vi "Flatten I2C Linux Header.vi"(8 "error in (no error)":errorcluster, 9 "Flattened Data in":u8[](array[numeric])=[0, 0, 0, 0, 0, 0, 0, 0] format="%.0x", 10 "I2C Linux Header in":T1, 11 "pcap Parse and Build in":refnum<class "pcap Parse and Build.lvclass">) -> (0 "error out":errorcluster, 1 "Flattened Data out":u8[](array[numeric])=[0, 0, 0, 0, 0, 0, 0, 0, 1, 2, 3, 4, 5], 2 "I2C Linux Header out":T1, 3 "pcap Parse and Build out":refnum<class "pcap Parse and Build.lvclass">)   [LabVIEW 2021, in "pcap Parse and Build.lvclass"]
uses:
  pcap Parse and Build.lvclass
  pcap Parse and Build.lvclass/pcap Parse and Build.ctl
  e4177ba7-55c0-4140-bea2-15e5e44a53d0.vi
  Typedef/I2C Linux Header.ctl
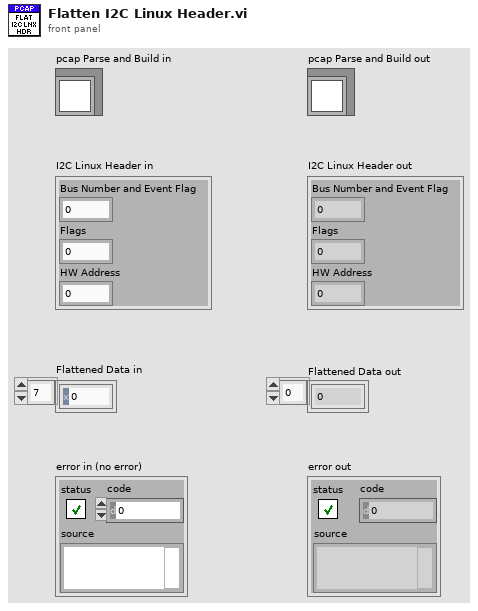
[diagram p1: front panel]
types:
  T1 = typedef "pcap Parse and Build.lvclass/I2C Linux Header.ctl" = cluster{"Bus Number and Event Flag":u8, "Flags":u32, "HW Address":u8}
  T2 = typedef "DataTypes_CIF_U.lvlib/Endian.ctl" = enum16{"Little Endian", "Big Endian"}
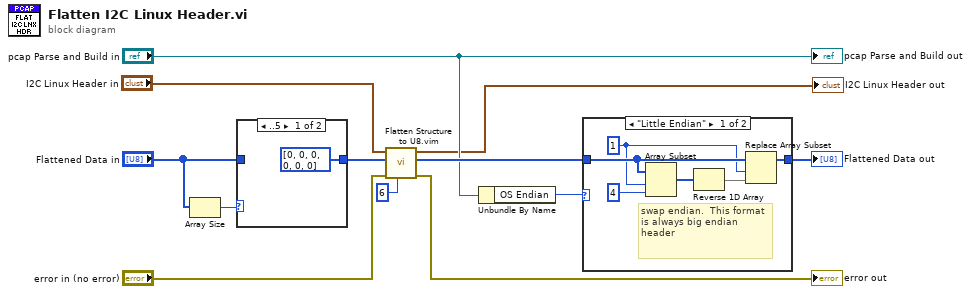
[diagram p0: block diagram]
diagram:
  n1 = Array Size(array="Flattened Data in") -> (size(s)=w8:i32)
  n2 = case shown="..5" w8 {
    tunnel: "Flattened Data in" -> [_ w14]
    tunnel: [u8[] [0, 0, 0, 0, 0, 0] ("Flattened Data in") w14] -> w9
    frame ..5 {
    }
    frame 6, Default {
    }
  }
  n3 = call "Flatten Structure to U8.vim"("Length override"=u64 6, "error in"="error in (no error)", "Flattened Data in"=w9, "Data to Flatten in"="I2C Linux Header in") -> ("error out"=→"error out":errorcluster, "Flattened Data out"=w7:u8[], "Data to Flatten out"=→"I2C Linux Header out":T1)  [unwired: 5 in]
  n4 = Unbundle By Name("pcap Parse and Build in") -> ("OS Endian"=w3:T2)
  n5 = case shown="\"Little Endian\"" w3 {
    tunnel: w7 -> [w18 w21]
    tunnel: [w16 w21] -> w6
    frame "Little Endian" {
      w15 = 1 ("index")
      # "swap endian.  This format is always big endian header"
      n6 = Array Subset(array=w18, index=w15, length=4 ("index")) -> (w19:u8[])
      n7 = Reverse 1D Array(array=w19) -> (reversed array=w17:u8[])
      n8 = Replace Array Subset(array=w18, new element=w17, index=w15) -> (w16:u8[])
    }
    frame "Big Endian" {
    }
  }
  "Flattened Data out" <- w6
  "pcap Parse and Build out" <- "pcap Parse and Build in"
